vi "遊戲成就.vi"() -> ()   [LabVIEW 2014]
panel:
  out "目前在骰子比大\n小中獲勝之次數":i32
  out "目前在骰寶\n中猜對之次數":i32
  out "目前在十八仔中\n擲出一色之次數":i32
  out "距離目標金額相差":i32
  in  "退出視窗":bool
  in  "查看":bool
  in  "查看":bool
  in  "查看":bool
  in  "查看":bool
  in  "查看":bool
  out "很大喔~":bool
  out "神準無比":bool
  out "一色狂徒":bool
  out "骰子賭爛":bool
  out "骰子賭聖":bool
  # "達到條件 : 賭金金額\n達到2000以上。"
  # "獲得條件:賭金金額\n歸零或為負數。"
  # "達到條件:在骰寶中\n累積猜中50次。"
  # "達到條件:在骰子比\n大小中累積獲勝50次"
  # "達到條件:在十八仔\n中骰出一色10次。"
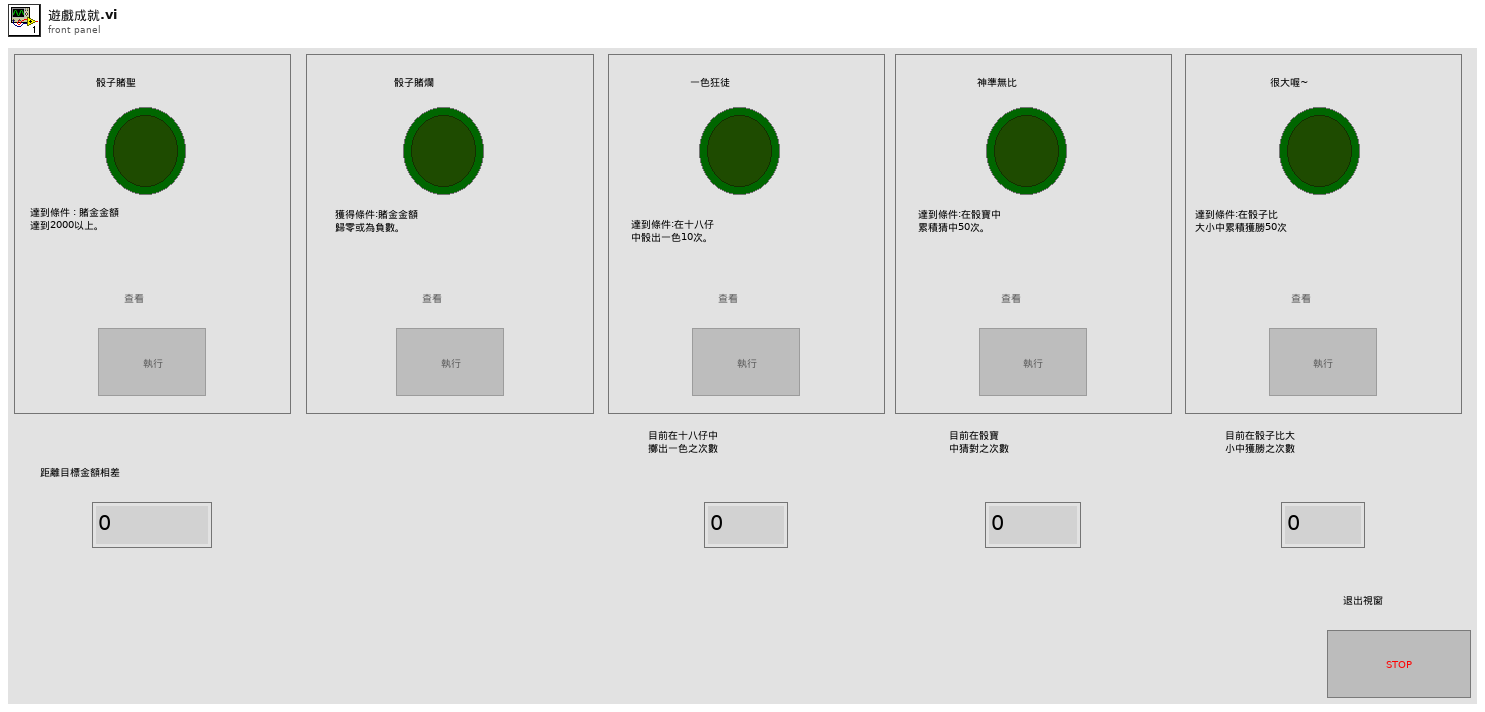
[diagram p1: front panel]
types:
  T1 = enum8{"Enabled", "Disabled", "Disabled and Grayed Out"}
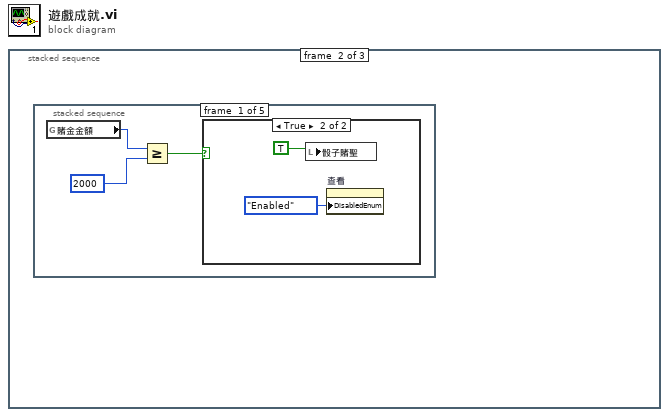
[diagram p0: block diagram]
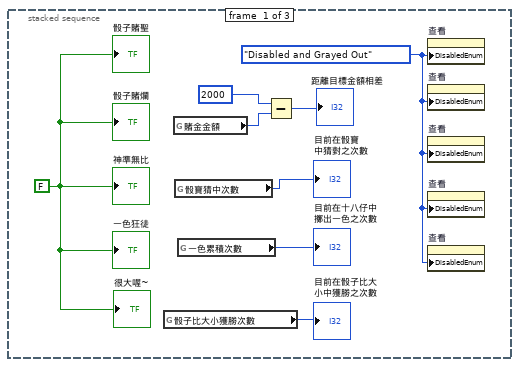
[diagram p2: hidden frame]
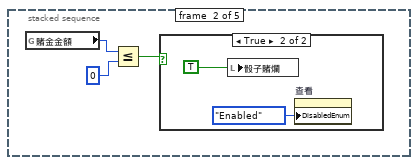
[diagram p4: hidden frame]
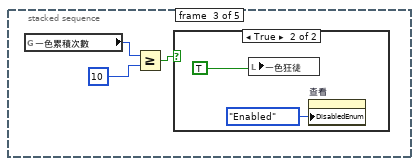
[diagram p6: hidden frame]
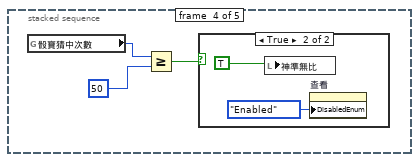
[diagram p8: hidden frame]
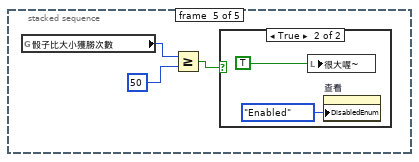
[diagram p10: hidden frame]
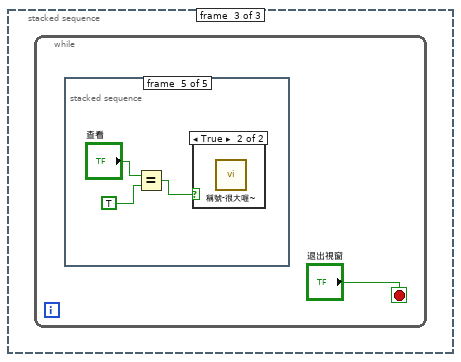
[diagram p12: hidden frame]
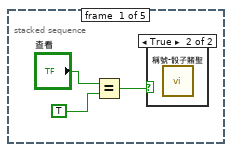
[diagram p13: hidden frame]
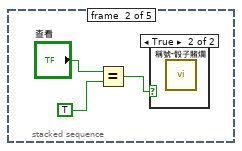
[diagram p15: hidden frame]
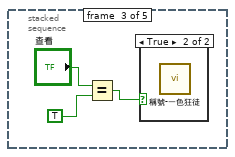
[diagram p17: hidden frame]
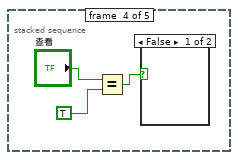
[diagram p19: hidden frame]
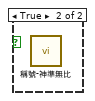
[diagram p20: hidden frame]
diagram:
  n1 = stacked-sequence {
    frame #0 {
      w7 = T1."Disabled and Grayed Out" ("Disabled")
      w8 = FALSE
      n2 = global read "global variable-骰子比大小獲勝次數.vi" "骰子比大小獲勝次數"() -> (→"目前在骰子比大\n小中獲勝之次數":i32)
      n3 = global read "global variable-賭金金額.vi" "賭金金額"() -> (w5:i32)
      n4 = global read "global variable-骰寶猜中次數.vi" "骰寶猜中次數"() -> (→"目前在骰寶\n中猜對之次數":i32)
      n5 = global read "global variable-一色累積次數.vi" "一色累積次數"() -> (→"目前在十八仔中\n擲出一色之次數":i32)
      n6 = Subtract(x=2000, y=w5) -> (x-y=→"距離目標金額相差":i32)
      n7 = property on="查看" class="Bool"("DisabledEnum"=w7) -> ()  [unwired: 2 in, 2 out]
      n8 = property on="查看" class="Bool"("DisabledEnum"=w7) -> ()  [unwired: 2 in, 2 out]
      n9 = property on="查看" class="Bool"("DisabledEnum"=w7) -> ()  [unwired: 2 in, 2 out]
      n10 = property on="查看" class="Bool"("DisabledEnum"=w7) -> ()  [unwired: 2 in, 2 out]
      n11 = property on="查看" class="Bool"("DisabledEnum"=w7) -> ()  [unwired: 2 in, 2 out]
      "骰子賭聖" <- w8
      "骰子賭爛" <- w8
      "一色狂徒" <- w8
      "神準無比" <- w8
      "很大喔~" <- w8
    }
    frame #1 {
      n12 = stacked-sequence {
        frame #0 {
          n13 = global read "global variable-賭金金額.vi" "賭金金額"() -> (w11:i32)
          n14 = Greater Or Equal?(x=w11, y=2000) -> (x >= y?=w9:bool)
          n15 = case shown="True" w9 {
            frame False {
            }
            frame True {
              n16 = local write "骰子賭聖"(TRUE) -> ()
              n17 = property on="查看" class="Bool"("DisabledEnum"=T1."Enabled" ("Disabled")) -> ()  [unwired: 2 in, 2 out]
            }
          }
        }
        frame #1 {
          n18 = global read "global variable-賭金金額.vi" "賭金金額"() -> (w16:i32)
          n19 = Less Or Equal?(x=w16, y=0) -> (x <= y?=w14:bool)
          n20 = case shown="True" w14 {
            frame False {
            }
            frame True {
              n21 = local write "骰子賭爛"(TRUE) -> ()
              n22 = property on="查看" class="Bool"("DisabledEnum"=T1."Enabled" ("Disabled")) -> ()  [unwired: 2 in, 2 out]
            }
          }
        }
        frame #2 {
          n23 = global read "global variable-一色累積次數.vi" "一色累積次數"() -> (w21:i32)
          n24 = Greater Or Equal?(x=w21, y=10) -> (x >= y?=w19:bool)
          n25 = case shown="True" w19 {
            frame False {
            }
            frame True {
              n26 = local write "一色狂徒"(TRUE) -> ()
              n27 = property on="查看" class="Bool"("DisabledEnum"=T1."Enabled" ("Disabled")) -> ()  [unwired: 2 in, 2 out]
            }
          }
        }
        frame #3 {
          n28 = global read "global variable-骰寶猜中次數.vi" "骰寶猜中次數"() -> (w26:i32)
          n29 = Greater Or Equal?(x=w26, y=50) -> (x >= y?=w24:bool)
          n30 = case shown="True" w24 {
            frame False {
            }
            frame True {
              n31 = local write "神準無比"(TRUE) -> ()
              n32 = property on="查看" class="Bool"("DisabledEnum"=T1."Enabled" ("Disabled")) -> ()  [unwired: 2 in, 2 out]
            }
          }
        }
        frame #4 {
          n33 = global read "global variable-骰子比大小獲勝次數.vi" "骰子比大小獲勝次數"() -> (w31:i32)
          n34 = Greater Or Equal?(x=w31, y=50) -> (x >= y?=w29:bool)
          n35 = case shown="True" w29 {
            frame False {
            }
            frame True {
              n36 = local write "很大喔~"(TRUE) -> ()
              n37 = property on="查看" class="Bool"("DisabledEnum"=T1."Enabled" ("Disabled")) -> ()  [unwired: 2 in, 2 out]
            }
          }
        }
      }
    }
    frame #2 {
      n38 = while {
        stop <- "退出視窗" stop-if-true
        n39 = stacked-sequence {
          frame #0 {
            n40 = Equal?(x="查看", y=TRUE) -> (x = y?=w37:bool)
            n41 = case shown="True" w37 {
              frame False {
              }
              frame True {
                n42 = call "稱號-骰子賭聖.vi"() -> ()  [unwired: 12 in]
              }
            }
          }
          frame #1 {
            n43 = Equal?(x="查看", y=TRUE) -> (x = y?=w40:bool)
            n44 = case shown="True" w40 {
              frame False {
              }
              frame True {
                n45 = call "稱號-骰子賭爛.vi"() -> ()  [unwired: 12 in]
              }
            }
          }
          frame #2 {
            n46 = Equal?(x="查看", y=TRUE) -> (x = y?=w43:bool)
            n47 = case shown="True" w43 {
              frame False {
              }
              frame True {
                n48 = call "稱號-一色狂徒.vi"() -> ()  [unwired: 12 in]
              }
            }
          }
          frame #3 {
            n49 = Equal?(x="查看", y=TRUE) -> (x = y?=w46:bool)
            n50 = case shown="False" w46 {
              frame False {
              }
              frame True {
                n51 = call "稱號-神準無比.vi"() -> ()  [unwired: 12 in]
              }
            }
          }
          frame #4 {
            n52 = Equal?(x="查看", y=TRUE) -> (x = y?=w49:bool)
            n53 = case shown="True" w49 {
              frame False {
              }
              frame True {
                n54 = call "稱號-很大喔~.vi"() -> ()  [unwired: 12 in]
              }
            }
          }
        }
      }
    }
  }
